vi "SENS_SEGM_FREQ_CENT.vi"(0 "VISA IN":refnum<visa-resource-name>, 1 "Segment":i32, 2 "Center Frq. (Hz)":i32, 5 "error in":errorcluster, 7 "Channel":i32) -> (14 "VISA Out":refnum<visa-resource-name>, 19 "error out":errorcluster)   [LabVIEW 2018, in "PNA-X.lvlib"]
doc: "SENSe<cnum>:SEGMent<snum>:FREQuency:CENTer <num> \n(Read-Write) Sets the Center Frequency for the specified segment. The Frequency Span of the \nsegment remains the same. The Start and Stop Frequencies change accordingly. \nNote: All previous segment's Start and Stop Frequencies that are larger than the new Start Frequency \nare changed to the new Start Frequency. All following segment's start and stop frequencies that are \nsmaller than the new Stop Frequency are changed to the new Stop Frequency. \nParameters \n<cnum> Any existing channel number. If unspecified, value is set to 1 \n<snum> Segment number to modify. Choose any existing segment number. \n<num> Center Frequency in Hz. Choose any number between the minimum and \nmaximum frequency of the analyzer. \nNote: This command will accept MIN or MAX instead of a numeric parameter. \nSee SCPI Syntax for more information. \nExamples SENS:SEGM:FREQ:CENT 1MHZ \nsense2:segment2:frequency:center 1e9 \nQuery Syntax SENSe<cnum>:SEGMent<snum>:FREQuency:CENTer? \nReturn Type Numeric \nDefault Stop Frequency of the previous segment. If first segment, start frequency of the \nanalyzer."
uses:
  PNA-X.lvlib
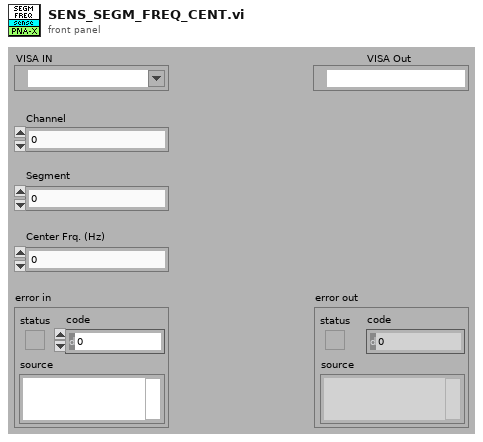
[diagram p1: front panel]
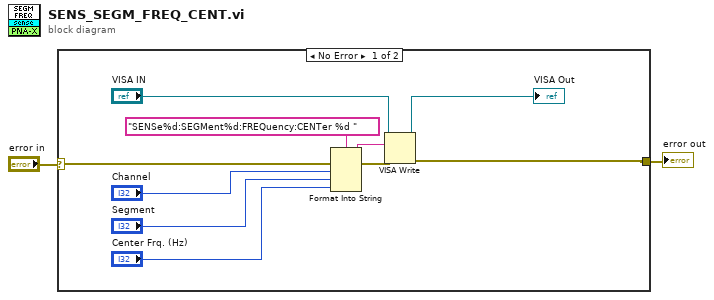
[diagram p0: block diagram]
diagram:
  n1 = case shown="No Error" "error in" {
    selector: "error in" -> [w12 w13]
    tunnel: [w7 w13] -> w1
    frame No Error {
      n2 = Format Into String(format string="SENSe%d:SEGMent%d:FREQuency:CENTer %d " ("Cmdline"), error in=w12, "Channel", "Segment", "Center Frq. (Hz)") -> (resulting string=w10:string, error out=w11:errorcluster)  [unwired: 1 in]
      n3 = VISA Write(VISA resource name="VISA IN", write buffer=w10, error in (no error)=w11) -> (VISA resource name out=→"VISA Out":refnum<visa-resource-name>, error out=w7:errorcluster)  [unwired: 1 out]
    }
    frame Error {
    }
  }
  "error out" <- w1
